vi "IR_READ_WRITE_v2.vi"(9 "IR Read Directory":string="C:\\Users\\Admin\\Documents\\Data\\Experiment 2016-02-27 15-03 MS IR Validation PS", 11 "Peaks":dbl[][](array[numeric])=[[1737.0, 1700.0, 1667.0]]) -> ()   [LabVIEW 2015]
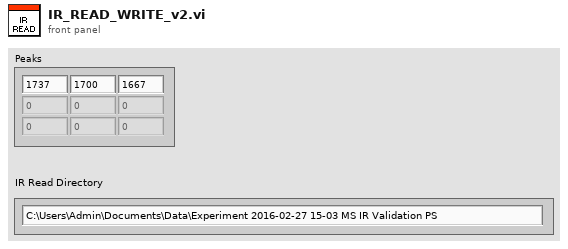
[diagram p1: front panel]
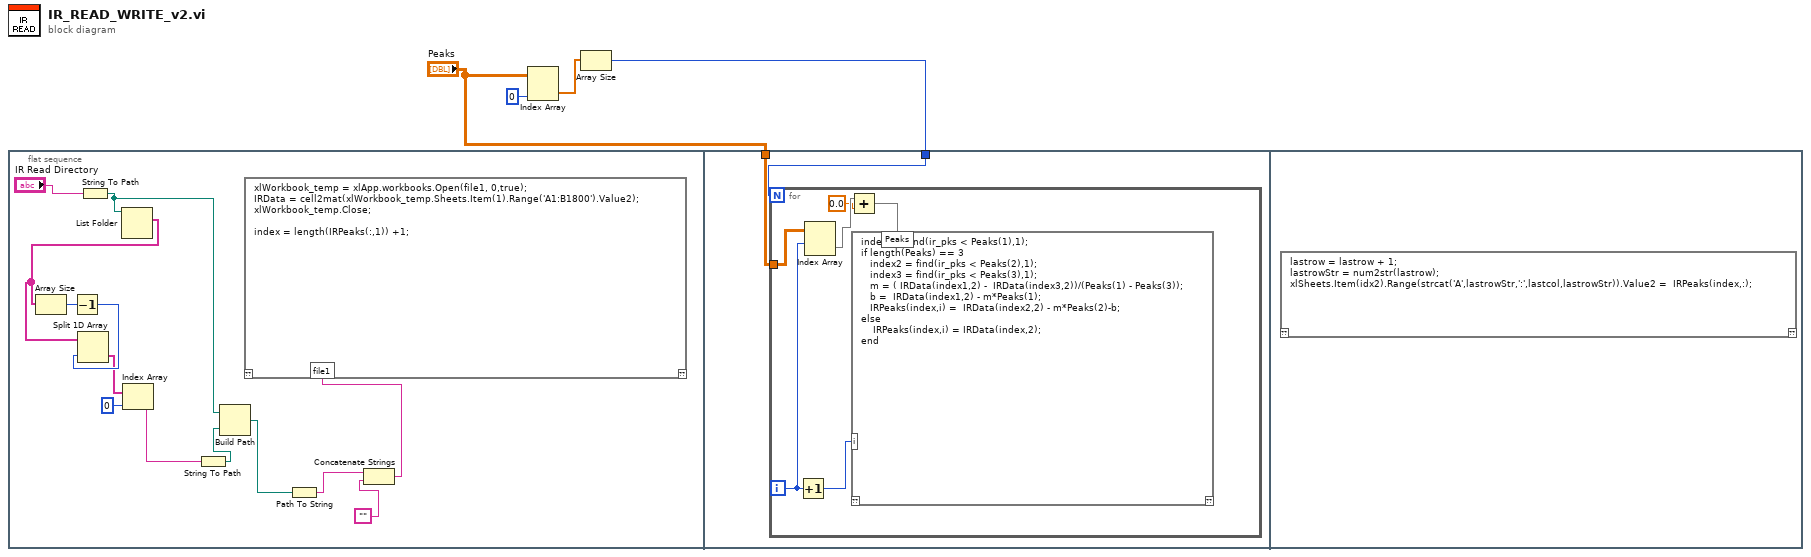
[diagram p0: block diagram]
diagram:
  n1 = flat-sequence {
    tunnel: "Peaks" -> [w19]
    tunnel: w1 -> [w18]
    frame #0 {
      n2 = String To Path(string="IR Read Directory") -> (path=w5:path)
      n3 = List Folder(path=w5) -> (filenames=w15:string[])  [unwired: 3 in, 3 out]
      n4 = Array Size(array=w15) -> (size(s)=w16:i32)
      n5 = Decrement(x=w16) -> (x-1=w14:i32)
      n6 = Split 1D Array(array=w15, index=w14) -> (second subarray=w13:string[])  [unwired: 1 out]
      n7 = Index Array(array=w13, index=0) -> (element=w10:string)
      n8 = String To Path(string=w10) -> (path=w11:path)
      n9 = Build Path(base path=w5, name or relative path=w11) -> (appended path=w7:path)
      n10 = Path To String(path=w7) -> (string=w9:string)
      n11 = Concatenate Strings(w9, "") -> (w6:string)
      n12 = script code="xlWorkbook_temp = xlApp.workbooks.Open(file1, 0,true);\nIRData = cell2mat(xlWorkbook_temp.Sheets.Item(1).Range('A1:B1800').Value2); \nxlWorkbook_temp.Close;\n\nindex = length(IRPeaks(:,1)) +1;"("file1"=w6) -> ()  [unwired: 1 in, 1 out]
    }
    frame #1 {
      n13 = for {
        N: w18 -> [_]
        tunnel: w19 -> [w24]
        i -> [w23]
        n14 = Increment(x=w23) -> (x+1=w25:i32)
        n15 = Index Array(array=w24, index (row)=w23) -> (element=w22:dbl[])  [unwired: 1 in]
        n16 = Add(x=w22, y=0.0) -> (x+y=w20:dbl[])
        n17 = script code="index1 = find(ir_pks < Peaks(1),1);\nif length(Peaks) == 3\n   index2 = find(ir_pks < Peaks(2),1);\n   index3 = find(ir_pks < Peaks(3),1);\n   m = ( IRData(index1,2) -  IRData(index3,2))/(Peaks(1) - Peaks(3));\n   b =  IRData(index1,2) - m*Peaks(1);\n   IRPeaks(index,i) =  IRData(index2,2) - m*Peaks(2)-b;\nelse\n    IRPeaks(index,i) = IRData(index,2);\nend"("i"=w25, "Peaks"=w20) -> ()  [unwired: 1 in, 1 out]
      }
    }
    frame #2 {
      n18 = script code="lastrow = lastrow + 1;\nlastrowStr = num2str(lastrow);\nxlSheets.Item(idx2).Range(strcat('A',lastrowStr,':',lastcol,lastrowStr)).Value2 =  IRPeaks(index,:);"() -> ()  [unwired: 1 in, 1 out]
    }
  }
  n19 = Index Array(array="Peaks", index (col)=0 ("disabled index (col)")) -> (element=w3:dbl[])  [unwired: 1 in]
  n20 = Array Size(array=w3) -> (size(s)=w1:i32)
